vi "NI VeriStand - Close Project Reference.vi"(8 "error in (no error)":errorcluster, 11 "Project Ref":T1) -> (0 "error out":errorcluster)   [LabVIEW 2020, in "NI_VS Project ExecutionAPI.lvlib"]
doc: "Closes an open reference to an NI VeriStand project."
uses:
  <vilib>/NI VeriStand/Execution/Project/NI_VS Project ExecutionAPI.lvlib
  <vilib>/NI VeriStand/Execution/Project/Project Ref.ctl
  NationalInstruments.VeriStand.ClientAPI
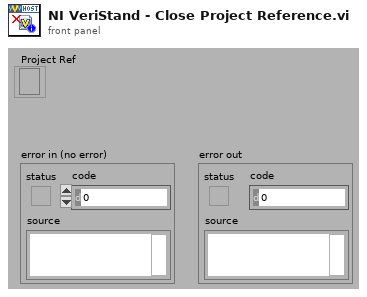
[diagram p1: front panel]
types:
  T1 = typedef "NI_VS Project ExecutionAPI.lvlib/Project Ref.ctl" = refnum<k24>
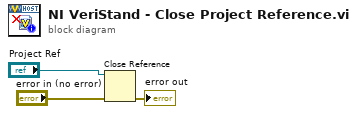
[diagram p0: block diagram]
diagram:
  n1 = Close Reference(reference="Project Ref", error in (no error)="error in (no error)") -> (error out=→"error out":errorcluster)
